vi "LcPictureBox_Create.vi"(0 "reference in":refnum<class "LcPictureBox.lvclass">, 2 "PictureBox":refnum<k24>, 3 "PictureBoxActiveXReference":refnum<vi>, 4 "BgColor(None)":u32(colorbox)=16777216, 5 "Error In":errorcluster, 6 "CacheNumberOfPensAndColors(0)":i32) -> (14 "reference out":refnum<class "LcPictureBox.lvclass">, 17 "ImageSizeUsed":cluster{"Width":i32, "Height":i32}, 19 "Error Out":errorcluster)   [LabVIEW 2020, in "LcPictureBox.lvclass"]
uses:
  LcPictureBox.lvclass
  System.Drawing
  SmoothingMode.ctl
  System.Windows.Forms
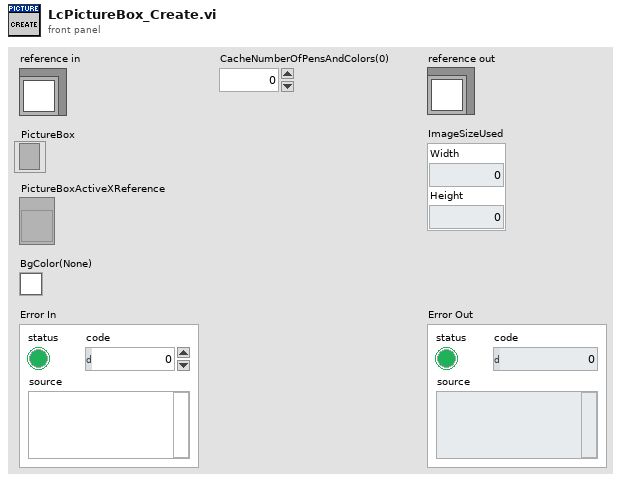
[diagram p1: front panel]
types:
  T1 = typedef "LcPictureBox.lvclass/SmoothingMode.ctl" = enum16{"None", "HighSpeed", "HighQuality", "AntiAlias"}
  T2 = typedef "LVBoundsTypeDef.ctl" = cluster{"Width":u32, "Height":u32}
  T3 = typedef "LcPictureBox.lvclass/ObjectAttributes.ctl" = cluster{"PictureBox":refnum<k24>, "ImageSize":cluster{"Width":i32, "Height":i32}, "PenMemory":map{cluster{"Alpha(100%)":dbl, "Color(Black)":u32, "Pen(Width=1, Solid)":T4}, refnum<k24>}, "GraphicsRef":refnum<k24>, "BrushMemory":map{cluster{"Alpha(100%)":dbl, "Color(Black)":u32}, refnum<k24>}, "Images":refnum<k24>[], "ImageIndex":i32, "BgColor(None)":u32, "LoadedImages":map{string, cluster{"ImageOut":refnum<k24>, "ImageSize":cluster{"Width":i32, "Height":i32}}}, "ColorsMemory":map{cluster{"Alpha(100%)":dbl, "Color(Black)":u32}, refnum<k24>}, "CacheSize":i32, "PictureBoxActiveXReference":refnum<vi>, "Scale":sgl, "Offset":cluster{"x":sgl, "y":sgl}, "zoom_center":cluster{"X":i32, "Y":i32}, "ImagesCreated":refnum<k24>[]}
  T4 = typedef "LcPictureBox.lvclass/Pen.ctl" = cluster{"Width":u16, "Style":enum32{"Solid", "Dash", "Dot", "DashDot", "DashDotDot"}}
  T5 = map{cluster{"Alpha(100%)":dbl, "Color(Black)":u32}, refnum<k24>}
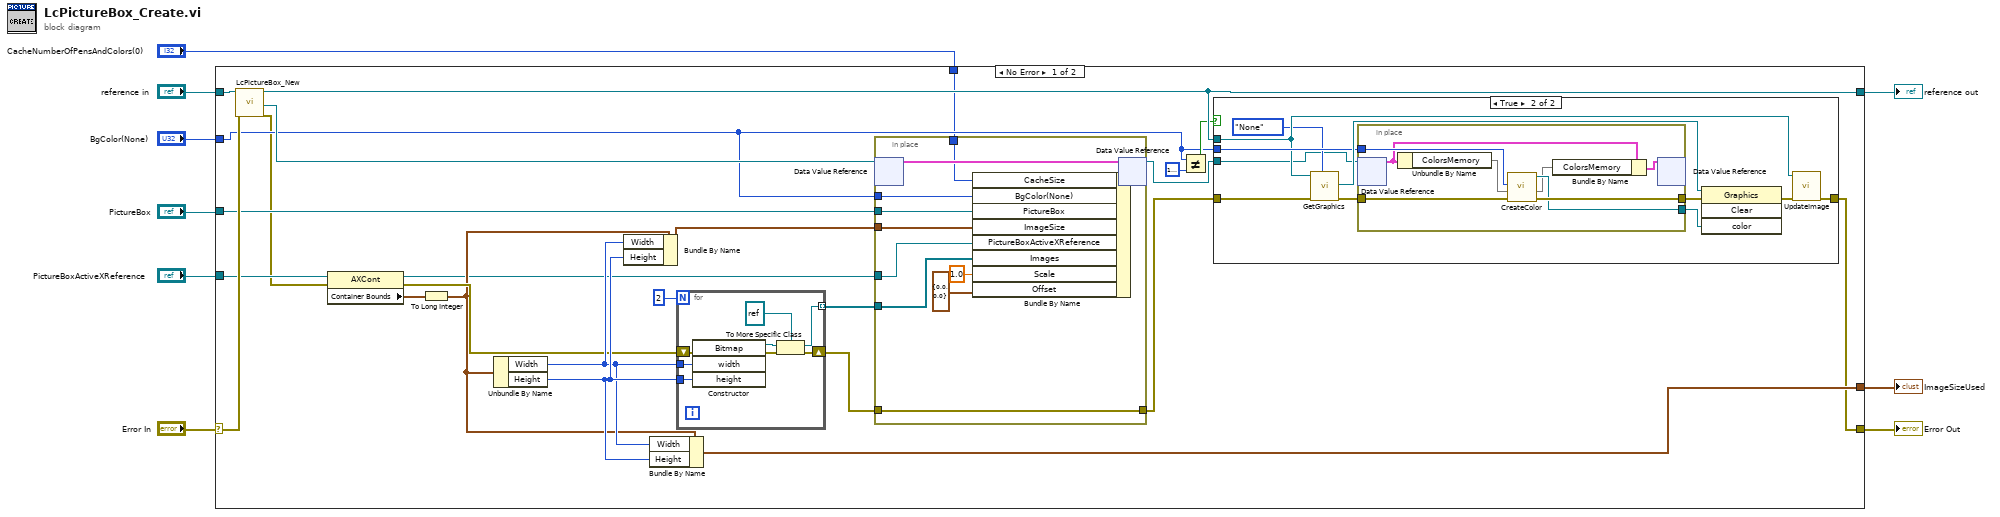
[diagram p0: block diagram]
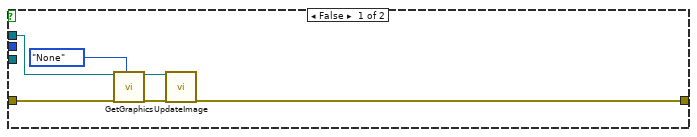
[diagram p2: hidden frame]
diagram:
  n1 = case shown="No Error" "Error In" {
    selector: "Error In" -> [w33 w80]
    tunnel: [w23 w80] -> w8
    tunnel: "reference in" -> [w34 w79]
    tunnel: [w24 w79] -> w6
    tunnel: "PictureBox" -> [w30 _]
    tunnel: [w26 _] -> w4
    tunnel: "BgColor(None)" -> [w20 _]
    tunnel: "CacheNumberOfPensAndColors(0)" -> [w16 _]
    tunnel: "PictureBoxActiveXReference" -> [w15 _]
    frame No Error {
      n2 = call "LcPictureBox_New.vi"("reference in"=w34, "error in (no error)"=w33) -> ("reference out"=w24:refnum<class "LcPictureBox.lvclass">, "DVRRefOut"=w32:refnum<data-value>, "error out"=w14:errorcluster)  [unwired: 14 in, 1 out]
      n3 = property class="AXCont"(reference=w15, error in=w14) -> (reference out=w10:refnum<vi>, error out=w13:errorcluster, "Container Bounds"=w12:T2)
      n4 = To Long Integer(number=w12) -> (32bit integer=w11:cluster{"Width":i32, "Height":i32})
      n5 = Unbundle By Name(w11) -> ("Width"=w18:i32, "Height"=w31:i32)
      n6 = Bundle By Name(cluster=w11, "Width"=w18, "Height"=w31) -> (w19:cluster{"Width":i32, "Height":i32})
      n7 = Bundle By Name(cluster=w11, "Width"=w18, "Height"=w31) -> (w26:cluster{"Width":i32, "Height":i32})
      n8 = for {
        N: 2 -> [_]
        tunnel: w18 -> [w65]
        tunnel: w31 -> [w64]
        shift-right: [w61] -> w29
        shift-left: w13 -> [w62]
        tunnel: [w60] -> w27 mode=indexing
        n9 = constructor class="Bitmap"(error in=w62, "width"=w65, "height"=w64) -> (reference out=w66:refnum<k24>, error out=w63:errorcluster)  [unwired: 2 in, 3 out]
        n10 = To More Specific Class(target class=refnum<k24> refnum, reference=w66, error in=w63) -> (specific class reference=w60:refnum<k24>, error out=w61:errorcluster)
      }
      n11 = in-place {
        in-place-border: w29 -> [w76]
        in-place-border: [w76] -> w21
        in-place-border: w30 -> [w75]
        in-place-border: w19 -> [w74]
        in-place-border: w27 -> [w71]
        in-place-border: w20 -> [w73]
        in-place-border: w16 -> [w72]
        in-place-border: w10 -> [w70]
        n12 = in-place-dvr #1(w32) -> (w77:T3)  [unwired: 1 out]
        n13 = Bundle By Name(cluster=w77, "CacheSize"=w72, "BgColor(None)"=w73, "PictureBox"=w75, "ImageSize"=w74, "PictureBoxActiveXReference"=w70, "Images"=w71, "Scale"=sgl 1.0 ("ScaleFactor(1)"), "Offset"=cluster{"x":sgl, "y":sgl} {"x"=0.0, "y"=0.0} ("UpperLeftCorner")) -> (w78:T3)
        n14 = in-place-dvr #1(w78) -> (w17:refnum<data-value>)  [unwired: 1 out]
      }
      n15 = Not Equal?(x=w20, y=u32 16777216 ("BgColor(None)")) -> (x != y?=w22:bool)
      n16 = case shown="True" w22 {
        tunnel: w20 -> [_ w50]
        tunnel: w24 -> [w39 w47]
        tunnel: [w40 w46] -> w23
        tunnel: w21 -> [w38 w45]
        tunnel: w17 -> [_ w41]
        frame False {
          n17 = call "GetGraphics.vi"("LcPictureBox in"=w39, "error in (no error)"=w38, "SmoothingMode"=SmoothingMode."None") -> ("LcPictureBox out"=w37:refnum<class "LcPictureBox.lvclass">, "error out"=w36:errorcluster)  [unwired: 12 in, 3 out]
          n18 = call-dynamic "UpdateImage.vi"("reference in"=w37, "Error In"=w36) -> ("Error Out"=w40:errorcluster)  [unwired: 14 in, 3 out]
        }
        frame True {
          n19 = call "GetGraphics.vi"("LcPictureBox in"=w47, "error in (no error)"=w45, "SmoothingMode"=SmoothingMode."None") -> ("Graphics"=w51:refnum<k24>, "error out"=w49:errorcluster)  [unwired: 12 in, 3 out]
          n20 = in-place {
            in-place-border: w50 -> [w59]
            in-place-border: w49 -> [w58]
            in-place-border: [w57] -> w48
            in-place-border: [w56] -> w42
            n21 = in-place-dvr #2(w41) -> (w54:T3)  [unwired: 1 out]
            n22 = Unbundle By Name(w54) -> ("ColorsMemory"=w55:T5)
            n23 = call "CreateColor.vi"("error in (no error)"=w58, "ColorsIn"=w55, "Color(Black)"=w59) -> ("error out"=w57:errorcluster, "ColorsOut"=w53:T5, "ColorRef"=w56:refnum<k24>)  [unwired: 6 in]
            n24 = Bundle By Name(cluster=w54, "ColorsMemory"=w53) -> (w52:T3)
            n25 = in-place-dvr #2(w52) -> ()  [unwired: 2 out]
          }
          n26 = invoke class="Graphics" method="Clear"(reference=w51, error in=w48, "color"=w42) -> (error out=w43:errorcluster)  [unwired: 1 in, 3 out]
          n27 = call-dynamic "UpdateImage.vi"("reference in"=w47, "Error In"=w43) -> ("Error Out"=w46:errorcluster)  [unwired: 14 in, 3 out]
        }
      }
    }
    frame Error {
      # "VI-TechBaseTemplate_Simple_4x4x4"
    }
  }
  "Error Out" <- w8
  "reference out" <- w6
  "ImageSizeUsed" <- w4
